vi "Send Validate Response.vi"(7 "Message Priority (Normal)":T2=enum."Normal", 8 "error in (no error)":errorcluster, 10 "Response Data":T1, 11 "Message Enqueuer":refnum<class "Message Enqueuer.lvclass">) -> (0 "error out":errorcluster, 3 "Message Enqueuer out":refnum<class "Message Enqueuer.lvclass">)   [LabVIEW 2017, in "Text based Communications Test.lvlib" / "Validate Response Msg.lvclass"]
doc: "This VI sends the message to an actor."
uses:
  Validate Response Msg.lvclass
  <vilib>/ActorFramework/Message Enqueuer/Message Enqueuer.lvclass
  <vilib>/ActorFramework/Message Enqueuer/Message Priority.ctl
  Text based Communications Test/File Data Format.ctl
  C:/Program Files (x86)/National Instruments/LabVIEW 2017/vi.lib/ActorFramework/Message/Message.lvclass
  Validate Response Msg.lvclass/Validate Response Msg.ctl
  <vilib>/ActorFramework/Message Enqueuer/Message Enqueuer.lvclass/Message Enqueuer.ctl
  <vilib>/ActorFramework/Message Priority Queue/Priority Enqueue.vi
  Text based Communications Test/Text based Communications Test.lvlib
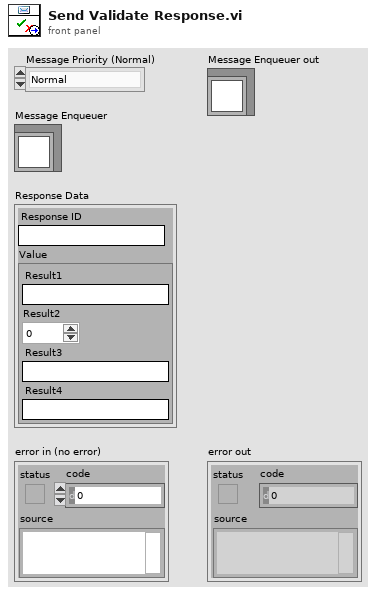
[diagram p1: front panel]
types:
  T1 = typedef "Text based Communications Test.lvlib/File Data Format.ctl" = cluster{"Response ID":string, "Value":cluster{"Result1":string, "Result2":dbl, "Result3":string, "Result4":string}}
  T2 = typedef "Actor Framework.lvlib/Message Enqueuer.lvclass/Message Priority.ctl" = enum16{"Low", "Normal", "High"}
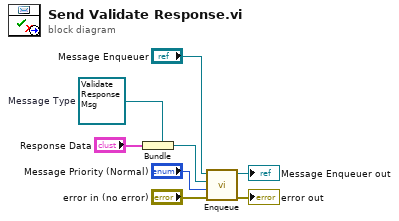
[diagram p0: block diagram]
diagram:
  w5 = refnum<class "Validate Response Msg.lvclass"> refnum  # Message Type
  n1 = Bundle(cluster=w5, "Response Data") -> (w4:refnum<class "Validate Response Msg.lvclass">)
  n2 = call <vilib>:"Enqueue.vi"("error in (no error)"="error in (no error)", "Message Priority (Normal)"="Message Priority (Normal)", "Message"=w4, "Message Enqueuer in"="Message Enqueuer") -> ("error out"=→"error out":errorcluster, "Message Enqueuer out"=→"Message Enqueuer out":refnum<class "Message Enqueuer.lvclass">)  [unwired: 6 in]
